vi "Project.SilentDisconnect.vi"(9 "Undeploy System Definition (F)":bool, 10 "Password (\"\")":string, 11 "Gateway IP Address (\"\": localhost)":string) -> (0 "error out":errorcluster)   [LabVIEW 2013, in "MiscHelperVIs.lvlib"]
uses:
  MiscHelperVIs.lvlib
  <vilib>/NI Veristand/Execution/Workspace/NI_VS Workspace ExecutionAPI.lvlib
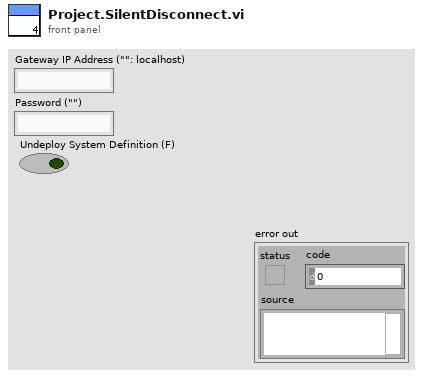
[diagram p1: front panel]
types:
  T1 = typedef "NI_VS Workspace ExecutionAPI.lvlib/WorkspaceAPI.ctl" = refnum<k24>
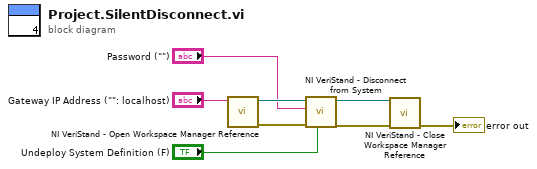
[diagram p0: block diagram]
diagram:
  n1 = call <vilib>:"NI VeriStand - Open Workspace Manager Reference.vi"("Gateway IP Address (\"\": localhost)"="Gateway IP Address (\"\": localhost)") -> ("error out"=w8:errorcluster, "WorkspaceManager"=w6:T1)  [unwired: 9 in]
  n2 = call <vilib>:"NI VeriStand - Disconnect from System.vi"("Undeploy System Definition (F)"="Undeploy System Definition (F)", "error in (no error)"=w8, "Password (\"\")"="Password (\"\")", "WorkspaceManager in"=w6) -> ("error out"=w3:errorcluster, "WorkspaceManager out"=w2:T1)  [unwired: 6 in]
  n3 = call <vilib>:"NI VeriStand - Close Workspace Manager Reference.vi"("error in (no error)"=w3, "WorkspaceManager"=w2) -> ("error out"=→"error out":errorcluster)  [unwired: 9 in]
